vi "WaveGeneratorSubV2.vi"(0 "Amplitude":dbl, 1 "Wave":T1 items=["0指令", "正弦波", "方波", "三角波", "常值", "波形数据", "白噪声", "正弦扫频", "梯度加载", "VMIC"], 2 "ForceSample":dbl format="%#_13g", 3 "Data array":dbl[](array[numeric]), 5 "Frequent":dbl, 7 "Angle":dbl, 9 "Offset":dbl, 11 "deltaF":dbl, 12 "VMIC":dbl format="%#_13g", 13 "dt":dbl, 14 "TestLoops":i32) -> (4 "Output":dbl, 10 "Output 2":dbl, 15 "waveout 3":dbl)   [LabVIEW 2020]
uses:
  WaveType.ctl
panel:
  in  "数值":i32
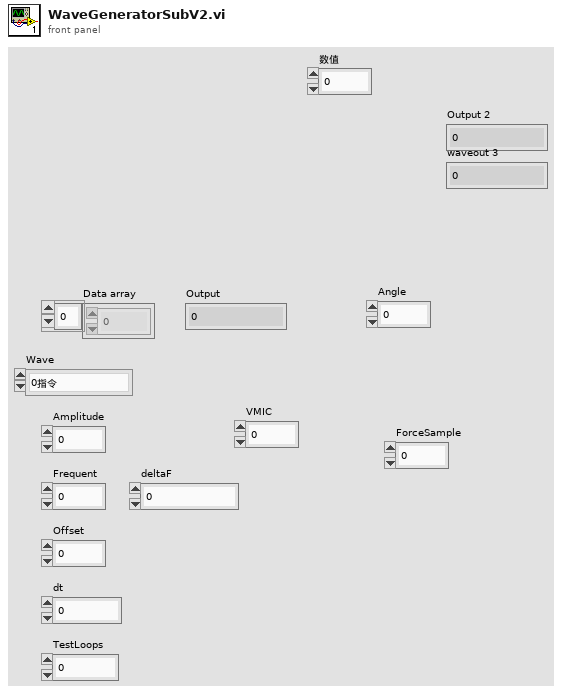
[diagram p1: front panel]
types:
  T1 = typedef "WaveType.ctl" = i32
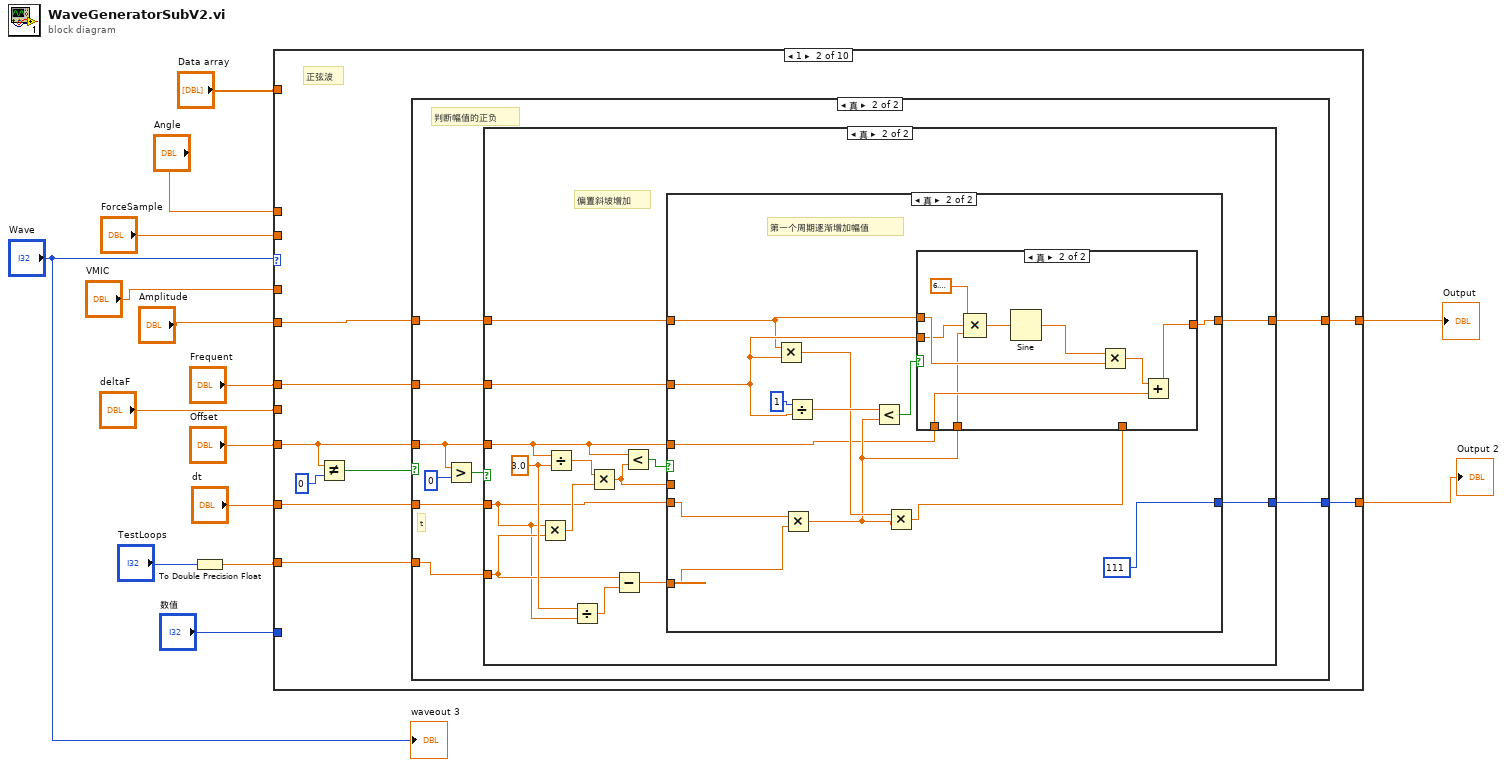
[diagram p0: block diagram]
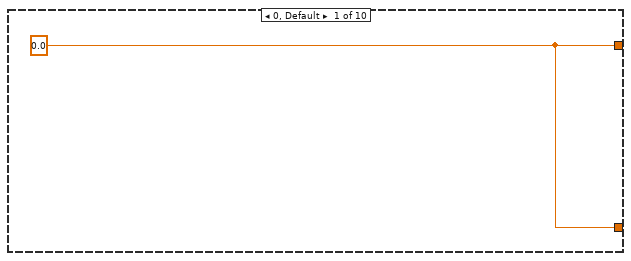
[diagram p2: hidden frame]
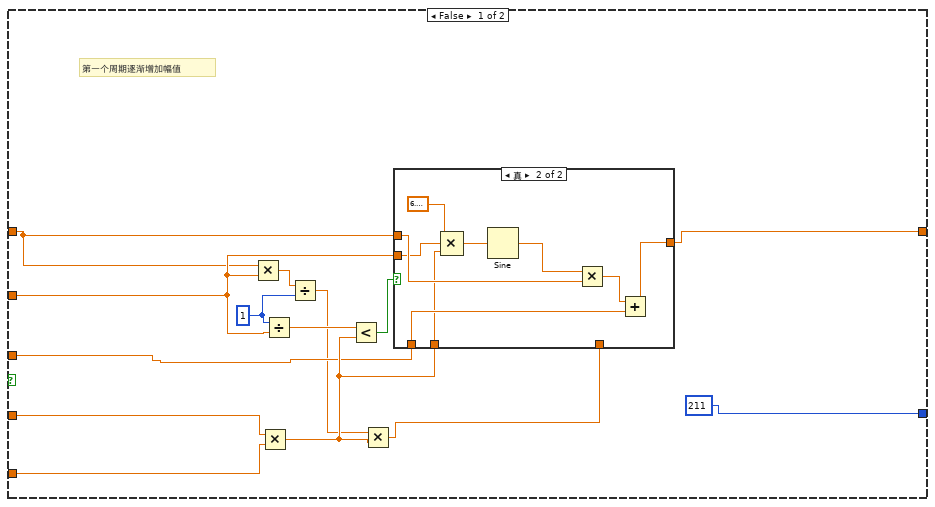
[diagram p3: hidden frame]
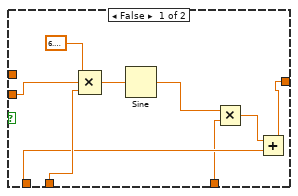
[diagram p4: hidden frame]
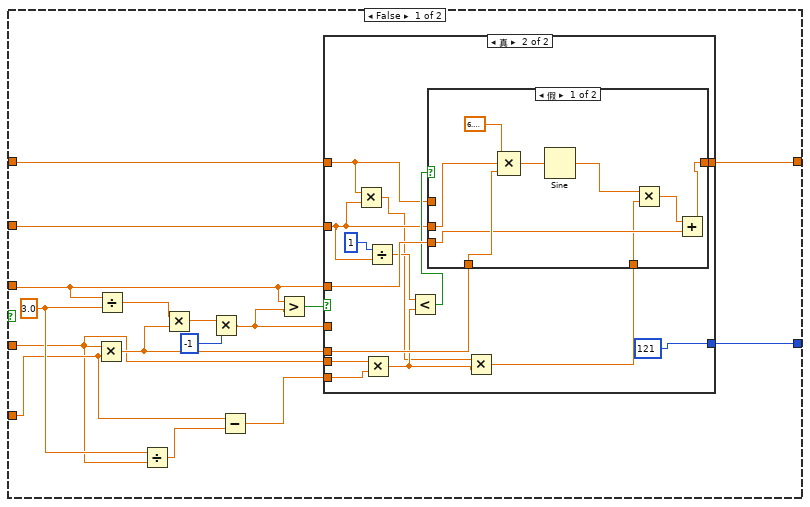
[diagram p5: hidden frame]
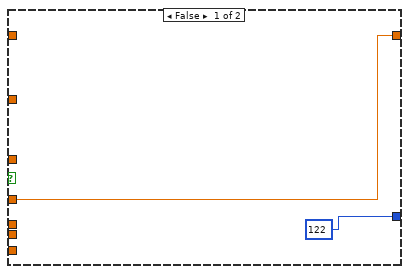
[diagram p6: hidden frame]
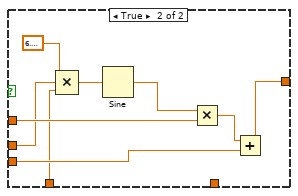
[diagram p7: hidden frame]
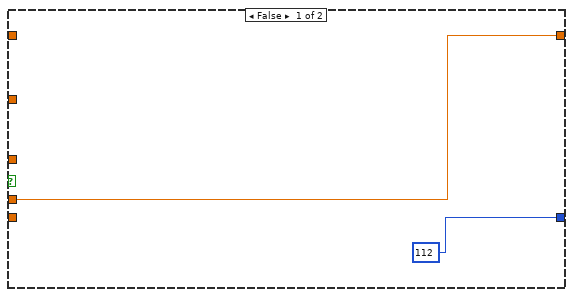
[diagram p8: hidden frame]
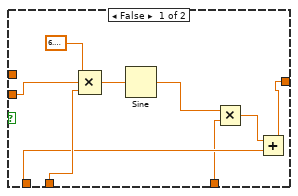
[diagram p9: hidden frame]
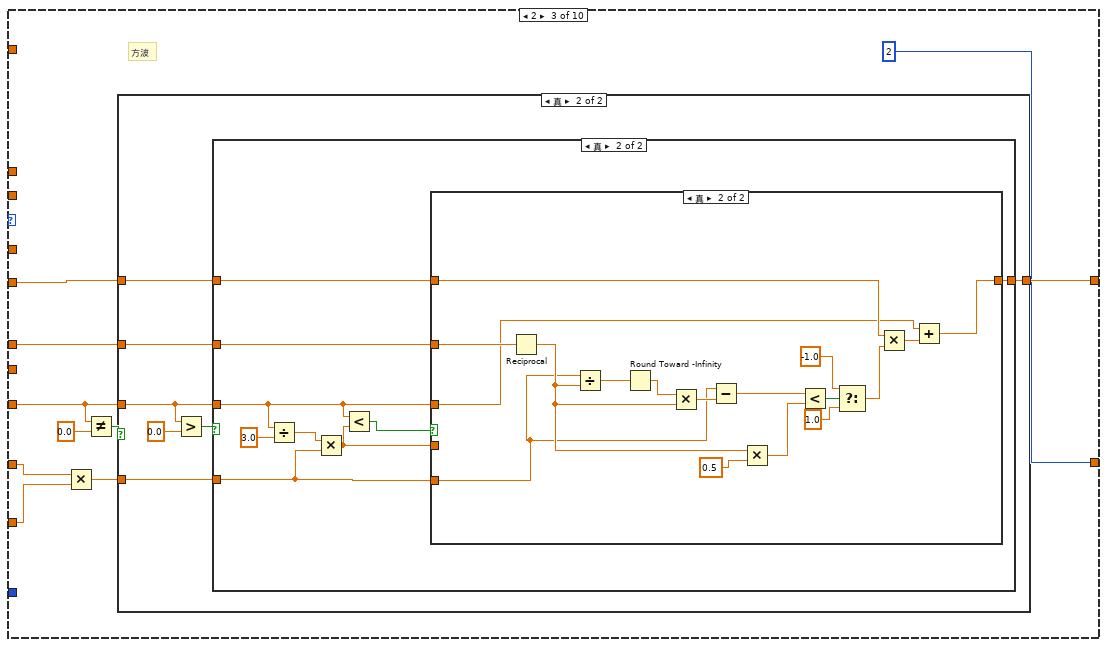
[diagram p10: hidden frame]
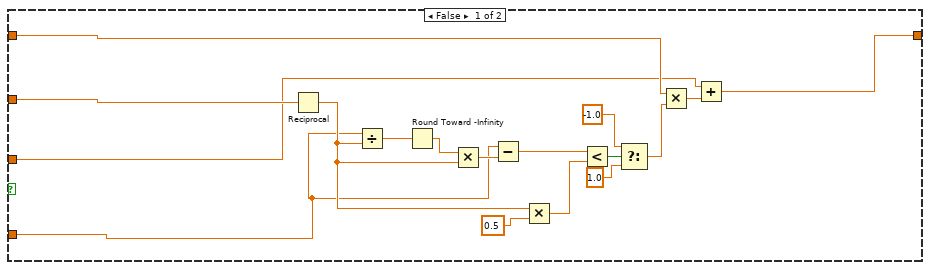
[diagram p11: hidden frame]
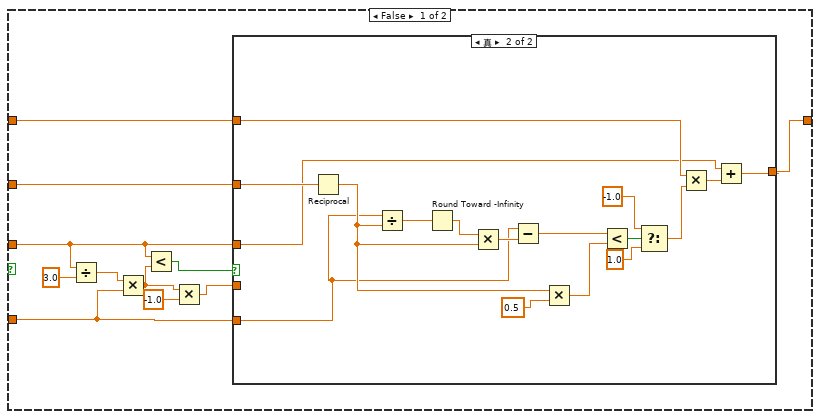
[diagram p12: hidden frame]
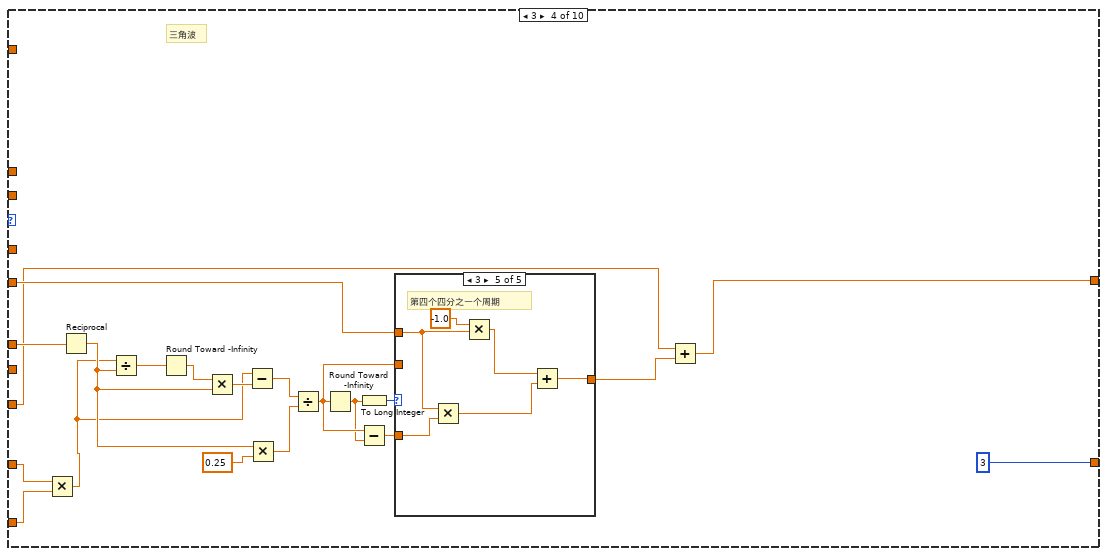
[diagram p15: hidden frame]
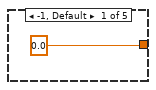
[diagram p16: hidden frame]
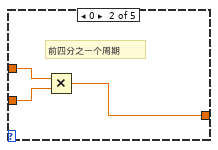
[diagram p17: hidden frame]
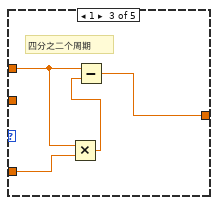
[diagram p18: hidden frame]
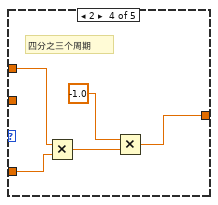
[diagram p19: hidden frame]
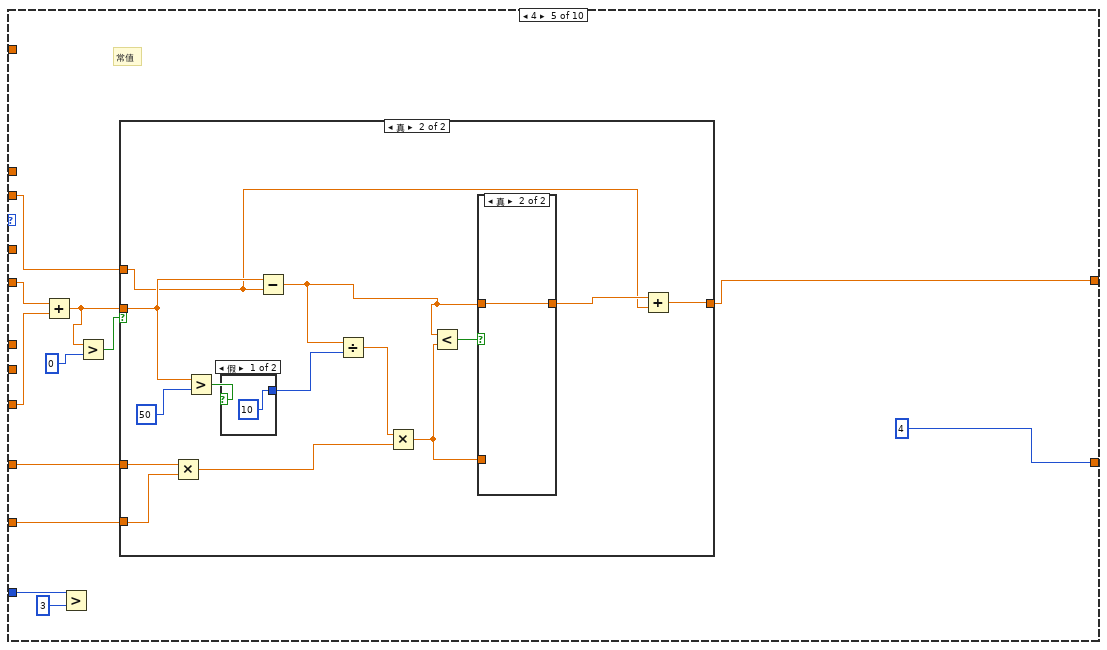
[diagram p20: hidden frame]
diagram:
  n1 = To Double Precision Float(number="TestLoops") -> (double precision float=w9:dbl)
  n2 = case shown="1" "Wave" {
    tunnel: "dt" -> [_ w21 w169 w257 w301 _ _ w362 _ _]
    tunnel: "Amplitude" -> [_ w24 w172 w265 w304 _ w351 w363 w372 _]
    tunnel: "Frequent" -> [_ w25 w173 w273 _ _ _ w356 _ _]
    tunnel: "Offset" -> [_ w18 w167 w259 w303 _ w344 w360 _ _]
    tunnel: "Data array" -> [_ _ _ _ _ w341 _ _ _ _]
    tunnel: w9 -> [_ w22 w170 w256 w302 w340 _ w358 _ _]
    tunnel: "deltaF" -> [_ _ _ _ _ _ _ w359 _ _]
    tunnel: "Angle" -> [_ _ _ _ _ _ _ _ w371 _]
    tunnel: [w16 w17 2 3 4 5 6 7 8 9] -> w7
    tunnel: "VMIC" -> [_ _ _ _ _ _ _ _ _ w373]
    tunnel: [w16 w23 w171 w258 w294 w339 w343 w364 w370 w373] -> w3
    tunnel: "数值" -> [_ _ _ _ w296 _ _ _ _ _]
    tunnel: "ForceSample" -> [_ _ _ _ w293 _ _ _ _ _]
    frame 0, Default {
      w16 = 0.0
    }
    frame 1 {
      # "正弦波"
      n3 = Not Equal?(x=w18, y=0) -> (x != y?=w19:bool)
      n4 = case shown="真" w19 {
        tunnel: w25 -> [w31 w66]
        tunnel: w24 -> [w30 w65]
        tunnel: [w35 w64] -> w23
        tunnel: w22 -> [w34 w63]
        tunnel: w21 -> [w33 w62]
        tunnel: w18 -> [w32 w59]
        tunnel: [211 w58] -> w17
        frame False {
          w28 = 1
          # "第一个周期逐渐增加幅值"
          n5 = Multiply(x=w30, y=w31) -> (x*y=w27:dbl)
          n6 = Multiply(x=w33, y=w34) -> (x*y=w36:dbl)
          n7 = Divide(x=w28, y=w31) -> (x/y=w39:dbl)
          n8 = Divide(x=w27, y=w28) -> (x/y=w26:dbl)
          n9 = Less?(x=w39, y=w36) -> (x < y?=w38:bool)
          n10 = Multiply(x=w26, y=w36) -> (x*y=w37:dbl)
          n11 = case shown="真" w38 {
            tunnel: w30 -> [_ w55]
            tunnel: w32 -> [w42 w53]
            tunnel: [w44 w51] -> w35
            tunnel: w36 -> [w43 w50]
            tunnel: w31 -> [w41 w49]
            tunnel: w37 -> [w40 _]
            frame False {
              n12 = Compound Arithmetic op=MULTIPLY(6.283185307179586, w41, w43) -> (w45:dbl)
              n13 = Sine(x=w45) -> (sin(x)=w47:dbl)
              n14 = Multiply(x=w47, y=w40) -> (x*y=w46:dbl)
              n15 = Add(x=w46, y=w42) -> (x+y=w44:dbl)
            }
            frame True {
              n16 = Compound Arithmetic op=MULTIPLY(6.283185307179586, w49, w50) -> (w52:dbl)
              n17 = Sine(x=w52) -> (sin(x)=w56:dbl)
              n18 = Multiply(x=w56, y=w55) -> (x*y=w54:dbl)
              n19 = Add(x=w54, y=w53) -> (x+y=w51:dbl)
            }
          }
        }
        frame True {
          # "判断幅值的正负"
          # "t"
          n20 = Greater?(x=w59, y=0) -> (0:w60:bool)
          n21 = case shown="真" w60 {
            tunnel: w66 -> [w75 w130]
            tunnel: w65 -> [w77 w129]
            tunnel: [w76 w128] -> w64
            tunnel: w63 -> [w74 w120]
            tunnel: w62 -> [w73 w118]
            tunnel: w59 -> [w68 w124]
            tunnel: [w67 w117] -> w58
            frame False {
              w80 = 3.0 ("y")
              n22 = Multiply(x=w73, y=w74) -> (x*y=w79:dbl)
              n23 = Divide(x=w68, y=w80) -> (x/y=w78:dbl)
              n24 = Divide(x=w80, y=w73) -> (x/y=w81:dbl)
              n25 = Multiply(x=w78, y=w79) -> (x*y=w72:dbl)
              n26 = Multiply(x=w72, y=-1) -> (x*y=w69:dbl)
              n27 = Subtract(x=w74, y=w81) -> (x-y=w82:dbl)
              n28 = Greater?(x=w68, y=w69) -> (0:w70:bool)
              n29 = case shown="真" w70 {
                tunnel: w75 -> [_ w89]
                tunnel: w77 -> [_ w90]
                tunnel: w68 -> [_ w98]
                tunnel: [w84 w97] -> w76
                tunnel: w79 -> [_ w96]
                tunnel: w69 -> [w84 _]
                tunnel: w82 -> [_ w92]
                tunnel: w73 -> [_ w91]
                tunnel: [122 121] -> w67
                frame False {
                }
                frame True {
                  n30 = Multiply(x=w90, y=w89) -> (x*y=w87:dbl)
                  n31 = Multiply(x=w91, y=w92) -> (x*y=w88:dbl)
                  n32 = Divide(x=1, y=w89) -> (x/y=w94:dbl)
                  n33 = Less?(x=w94, y=w88) -> (x < y?=w93:bool)
                  n34 = Multiply(x=w87, y=w88) -> (x*y=w86:dbl)
                  n35 = case shown="假" w93 {
                    tunnel: w90 -> [_ w114]
                    tunnel: w98 -> [w101 w112]
                    tunnel: [w103 w110] -> w97
                    tunnel: w96 -> [w102 w109]
                    tunnel: w89 -> [w100 w108]
                    tunnel: w86 -> [w99 _]
                    frame False {
                      n36 = Compound Arithmetic op=MULTIPLY(6.283185307179586, w100, w102) -> (w104:dbl)
                      n37 = Sine(x=w104) -> (sin(x)=w106:dbl)
                      n38 = Multiply(x=w106, y=w99) -> (x*y=w105:dbl)
                      n39 = Add(x=w105, y=w101) -> (x+y=w103:dbl)
                    }
                    frame True {
                      n40 = Compound Arithmetic op=MULTIPLY(6.283185307179586, w108, w109) -> (w111:dbl)
                      n41 = Sine(x=w111) -> (sin(x)=w115:dbl)
                      n42 = Multiply(x=w115, y=w114) -> (x*y=w113:dbl)
                      n43 = Add(x=w113, y=w112) -> (x+y=w110:dbl)
                    }
                  }
                }
              }
            }
            frame True {
              w122 = 3.0 ("y")
              # "偏置斜坡增加"
              n44 = Multiply(x=w118, y=w120) -> (x*y=w126:dbl)
              n45 = Divide(x=w124, y=w122) -> (x/y=w127:dbl)
              n46 = Divide(x=w122, y=w118) -> (x/y=w121:dbl)
              n47 = Multiply(x=w127, y=w126) -> (x*y=w123:dbl)
              n48 = Subtract(x=w120, y=w121) -> (x-y=w119:dbl)
              n49 = Less?(x=w124, y=w123) -> (x < y?=w125:bool)
              n50 = case shown="真" w125 {
                tunnel: w130 -> [_ w135]
                tunnel: w129 -> [_ w134]
                tunnel: w124 -> [_ w136]
                tunnel: [w132 w139] -> w128
                tunnel: w123 -> [w132 _]
                tunnel: w119 -> [_ w138]
                tunnel: w118 -> [_ w137]
                tunnel: [112 111] -> w117
                frame False {
                }
                frame True {
                  # "第一个周期逐渐增加幅值"
                  n51 = Multiply(x=w134, y=w135) -> (x*y=w142:dbl)
                  n52 = Multiply(x=w137, y=w138) -> (x*y=w140:dbl)
                  n53 = Divide(x=1, y=w135) -> (x/y=w144:dbl)
                  n54 = Less?(x=w144, y=w140) -> (x < y?=w143:bool)
                  n55 = Multiply(x=w142, y=w140) -> (x*y=w141:dbl)
                  n56 = case shown="真" w143 {
                    tunnel: w134 -> [_ w161]
                    tunnel: w136 -> [w148 w159]
                    tunnel: [w150 w157] -> w139
                    tunnel: w140 -> [w149 w156]
                    tunnel: w135 -> [w147 w155]
                    tunnel: w141 -> [w146 _]
                    frame False {
                      n57 = Compound Arithmetic op=MULTIPLY(6.283185307179586, w147, w149) -> (w151:dbl)
                      n58 = Sine(x=w151) -> (sin(x)=w153:dbl)
                      n59 = Multiply(x=w153, y=w146) -> (x*y=w152:dbl)
                      n60 = Add(x=w152, y=w148) -> (x+y=w150:dbl)
                    }
                    frame True {
                      n61 = Compound Arithmetic op=MULTIPLY(6.283185307179586, w155, w156) -> (w158:dbl)
                      n62 = Sine(x=w158) -> (sin(x)=w162:dbl)
                      n63 = Multiply(x=w162, y=w161) -> (x*y=w160:dbl)
                      n64 = Add(x=w160, y=w159) -> (x+y=w157:dbl)
                    }
                  }
                }
              }
            }
          }
        }
      }
    }
    frame 2 {
      # "方波"
      n65 = Multiply(x=w169, y=w170) -> (x*y=w168:dbl)
      n66 = Not Equal?(x=w167, y=0.0) -> (x != y?=w165:bool)
      n67 = case shown="真" w165 {
        tunnel: w173 -> [w176 w197]
        tunnel: w172 -> [w177 w196]
        tunnel: [w174 w195] -> w171
        tunnel: w168 -> [w178 w194]
        tunnel: w167 -> [w175 w193]
        frame False {
          n68 = Reciprocal(x=w176) -> (1/x=w186:dbl)
          n69 = Divide(x=w178, y=w186) -> (x/y=w190:dbl)
          n70 = Round Toward -Infinity(1:w190) -> (0:w189:dbl)
          n71 = Multiply(x=w189, y=w186) -> (x*y=w188:dbl)
          n72 = Subtract(x=w178, y=w188) -> (x-y=w187:dbl)
          n73 = Multiply(x=w186, y=0.5) -> (x*y=w184:dbl)
          n74 = Less?(x=w187, y=w184) -> (x < y?=w183:bool)
          n75 = Select(t=-1.0, s=w183, f=1.0) -> (s? t:f=w180:dbl)
          n76 = Multiply(x=w177, y=w180) -> (x*y=w179:dbl)
          n77 = Add(x=w175, y=w179) -> (x+y=w174:dbl)
        }
        frame True {
          n78 = Greater?(x=w193, y=0.0) -> (0:w191:bool)
          n79 = case shown="真" w191 {
            tunnel: w197 -> [w203 w235]
            tunnel: w196 -> [w202 w234]
            tunnel: [w201 w233] -> w195
            tunnel: w194 -> [w205 w230]
            tunnel: w193 -> [w204 w227]
            frame False {
              n80 = Divide(x=w204, y=3.0) -> (x/y=w207:dbl)
              n81 = Multiply(x=w207, y=w205) -> (x*y=w199:dbl)
              n82 = Less?(x=w204, y=w199) -> (x < y?=w206:bool)
              n83 = Multiply(x=w199, y=-1.0) -> (x*y=w198:dbl)
              n84 = case shown="真" w206 {
                tunnel: w203 -> [_ w226]
                tunnel: w202 -> [_ w214]
                tunnel: w204 -> [_ w212]
                tunnel: [w209 w211] -> w201
                tunnel: w205 -> [_ w210]
                tunnel: w198 -> [w209 _]
                frame False {
                }
                frame True {
                  n85 = Reciprocal(x=w226) -> (1/x=w221:dbl)
                  n86 = Divide(x=w210, y=w221) -> (x/y=w225:dbl)
                  n87 = Round Toward -Infinity(1:w225) -> (0:w224:dbl)
                  n88 = Multiply(x=w224, y=w221) -> (x*y=w223:dbl)
                  n89 = Subtract(x=w210, y=w223) -> (x-y=w222:dbl)
                  n90 = Multiply(x=w221, y=0.5) -> (x*y=w219:dbl)
                  n91 = Less?(x=w222, y=w219) -> (x < y?=w218:bool)
                  n92 = Select(t=-1.0, s=w218, f=1.0) -> (s? t:f=w215:dbl)
                  n93 = Multiply(x=w214, y=w215) -> (x*y=w213:dbl)
                  n94 = Add(x=w212, y=w213) -> (x+y=w211:dbl)
                }
              }
            }
            frame True {
              n95 = Divide(x=w227, y=3.0) -> (x/y=w231:dbl)
              n96 = Multiply(x=w231, y=w230) -> (x*y=w228:dbl)
              n97 = Less?(x=w227, y=w228) -> (x < y?=w229:bool)
              n98 = case shown="真" w229 {
                tunnel: w235 -> [_ w253]
                tunnel: w234 -> [_ w241]
                tunnel: w227 -> [_ w239]
                tunnel: [w236 w238] -> w233
                tunnel: w230 -> [_ w237]
                tunnel: w228 -> [w236 _]
                frame False {
                }
                frame True {
                  n99 = Reciprocal(x=w253) -> (1/x=w248:dbl)
                  n100 = Divide(x=w237, y=w248) -> (x/y=w252:dbl)
                  n101 = Round Toward -Infinity(1:w252) -> (0:w251:dbl)
                  n102 = Multiply(x=w251, y=w248) -> (x*y=w250:dbl)
                  n103 = Subtract(x=w237, y=w250) -> (x-y=w249:dbl)
                  n104 = Multiply(x=w248, y=0.5) -> (x*y=w246:dbl)
                  n105 = Less?(x=w249, y=w246) -> (x < y?=w245:bool)
                  n106 = Select(t=-1.0, s=w245, f=1.0) -> (s? t:f=w242:dbl)
                  n107 = Multiply(x=w241, y=w242) -> (x*y=w240:dbl)
                  n108 = Add(x=w239, y=w240) -> (x+y=w238:dbl)
                }
              }
            }
          }
        }
      }
    }
    frame 3 {
      # "三角波"
      n109 = Multiply(x=w257, y=w256) -> (x*y=w255:dbl)
      n110 = Reciprocal(x=w273) -> (1/x=w268:dbl)
      n111 = Divide(x=w255, y=w268) -> (x/y=w272:dbl)
      n112 = Round Toward -Infinity(1:w272) -> (0:w271:dbl)
      n113 = Multiply(x=w271, y=w268) -> (x*y=w270:dbl)
      n114 = Subtract(x=w255, y=w270) -> (x-y=w264:dbl)
      n115 = Multiply(x=w268, y=0.25) -> (x*y=w267:dbl)
      n116 = Divide(x=w264, y=w267) -> (x/y=w263:dbl)
      n117 = Round Toward -Infinity(1:w263) -> (0:w262:dbl)
      n118 = To Long Integer(number=w262) -> (32bit integer=w266:i32)
      n119 = Subtract(x=w263, y=w262) -> (x-y=w261:dbl)
      n120 = case shown="3" w266 {
        tunnel: w265 -> [_ w277 w278 w285 w289]
        tunnel: [0.0 w275 w279 w282 w290] -> w260
        tunnel: w263 -> [_ w276 _ _ _]
        tunnel: w261 -> [_ _ w281 w286 w292]
        frame -1, Default {
        }
        frame 0 {
          # "前四分之一个周期"
          n121 = Multiply(x=w277, y=w276) -> (x*y=w275:dbl)
        }
        frame 1 {
          # "四分之二个周期"
          n122 = Multiply(x=w278, y=w281) -> (x*y=w280:dbl)
          n123 = Subtract(x=w278, y=w280) -> (x-y=w279:dbl)
        }
        frame 2 {
          # "四分之三个周期"
          n124 = Multiply(x=w285, y=w286) -> (x*y=w284:dbl)
          n125 = Multiply(x=-1.0, y=w284) -> (x*y=w282:dbl)
        }
        frame 3 {
          # "第四个四分之一个周期"
          n126 = Multiply(x=w289, y=w292) -> (x*y=w288:dbl)
          n127 = Multiply(x=-1.0, y=w289) -> (x*y=w287:dbl)
          n128 = Add(x=w287, y=w288) -> (x+y=w290:dbl)
        }
      }
      n129 = Add(x=w259, y=w260) -> (x+y=w258:dbl)
    }
    frame 4 {
      # "常值"
      n130 = Add(x=w304, y=w303) -> (x+y=w300:dbl)
      n131 = Greater?(x=w296, y=3) -> ()  [unwired: 1 out]
      n132 = Greater?(x=w300, y=0) -> (0:w298:bool)
      n133 = case shown="真" w298 {
        tunnel: [w311 w324] -> w294
        tunnel: w302 -> [w310 w332]
        tunnel: w301 -> [w309 w331]
        tunnel: w300 -> [w308 w322]
        tunnel: w293 -> [_ w320]
        frame False {
          # "斜坡速率"
          n134 = Multiply(x=w309, y=w310) -> (x*y=w305:dbl)
          n135 = Less?(x=w308, y=-50) -> (x < y?=w307:bool)
          n136 = case shown="真" w307 {
            tunnel: [10 10] -> w314
            frame False {
            }
            frame True {
            }
          }
          n137 = Divide(x=w308, y=w314) -> (x/y=w312:dbl)
          n138 = Multiply(x=w312, y=w305) -> (x*y=w313:dbl)
          n139 = Greater?(x=w308, y=w313) -> (0:w315:bool)
          n140 = case shown="真" w315 {
            tunnel: w308 -> [_ w319]
            tunnel: [w318 w319] -> w311
            tunnel: w313 -> [w318 _]
            frame False {
            }
            frame True {
            }
          }
        }
        frame True {
          n141 = Multiply(x=w331, y=w332) -> (x*y=w329:dbl)
          n142 = Greater?(x=w322, y=50) -> (0:w325:bool)
          n143 = case shown="假" w325 {
            tunnel: [10 10] -> w330
            frame False {
            }
            frame True {
            }
          }
          n144 = Subtract(x=w322, y=w320) -> (x-y=w321:dbl)
          n145 = Divide(x=w321, y=w330) -> (x/y=w327:dbl)
          n146 = Multiply(x=w327, y=w329) -> (x*y=w328:dbl)
          n147 = Less?(x=w321, y=w328) -> (x < y?=w333:bool)
          n148 = case shown="真" w333 {
            tunnel: w321 -> [_ w337]
            tunnel: [w336 w337] -> w323
            tunnel: w328 -> [w336 _]
            frame False {
            }
            frame True {
            }
          }
          n149 = Add(x=w323, y=w320) -> (x+y=w324:dbl)
        }
      }
    }
    frame 5 {
      # "波形数据"
      n150 = Index Array(array=w341, index=w340) -> (element=w339:dbl)
    }
    frame 6 {
      # "白噪声"
      n151 = Random Number (0-1)() -> (number: 0 to 1=w350:dbl)
      n152 = Subtract(x=w350, y=0.5) -> (x-y=w348:dbl)
      n153 = Multiply(x=w348, y=w351) -> (x*y=w347:dbl)
      n154 = Multiply(x=w347, y=2.0) -> (x*y=w345:dbl)
      n155 = Add(x=w344, y=w345) -> (x+y=w343:dbl)
    }
    frame 7 {
      # "正弦扫频"
      n156 = Multiply(x=w362, y=w358) -> (x*y=w361:dbl)
      n157 = Multiply(x=w359, y=w358) -> (x*y=w357:dbl)
      n158 = Add(x=w356, y=w357) -> (x+y=w354:dbl)
      n159 = Multiply(x=0.5, y=w354) -> (x*y=w352:dbl)
      n160 = Compound Arithmetic op=MULTIPLY(6.283185307179586, w352, w361) -> (w365:dbl)
      n161 = Sine(x=w365) -> (sin(x)=w367:dbl)
      n162 = Multiply(x=w367, y=w363) -> (x*y=w366:dbl)
      n163 = Add(x=w366, y=w360) -> (x+y=w364:dbl)
    }
    frame 8 {
      # "梯度加载"
      n164 = Multiply(x=w371, y=w372) -> (x*y=w370:dbl)
    }
    frame 9 {
      # "VMIC"
    }
  }
  "Output" <- w3
  "Output 2" <- w7
  "waveout 3" <- "Wave"
